vi "Get Display Data.vi"(7 "Filter Configuration Array":refnum<class "Base Filter.lvclass">[](array[class]), 8 "error in (no error)":errorcluster, 11 "Standard Display Configuration in":refnum<class "Standard Display Configuration.lvclass">) -> (0 "error out":errorcluster, 2 "Display Data":T1)   [LabVIEW 2018, in "Assert API Components.lvlib" / "Assert Display.lvlib" / "Main Display.lvlib" / "Standard Display Configuration.lvclass"]
uses:
  Standard Display Configuration.lvclass
  C:/Users/UKHornP/Documents/Work/Projects/Assert API/Core/Main Display/Display Configurations/Base Display Configuration.lvclass
  Components/Display Data.ctl
  Main Display/Display Colours.ctl
  Assert API Components/Filter Configurations/Base Filter.lvclass
  Base Display Configuration.lvclass/Base Display Configuration.ctl
  Base Display Configuration.lvclass
  Main Display.lvlib
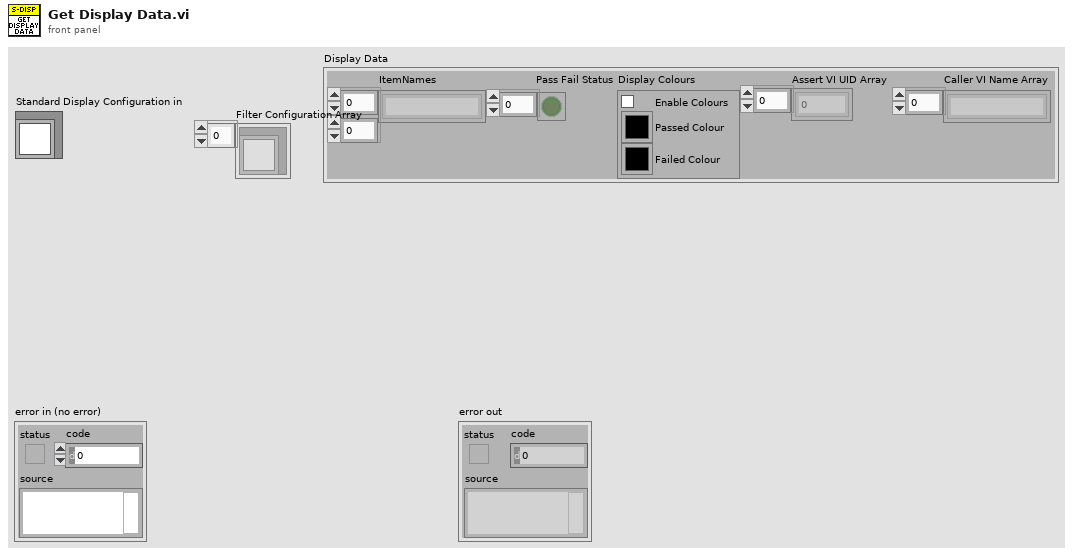
[diagram p1: front panel]
types:
  T1 = typedef "Assert API Components.lvlib/Assert Display.lvlib/Main Display.lvlib/Display Data.ctl" = cluster{"ItemNames":string[][], "Pass Fail Status":bool[], "Display Colours":T2, "Assert VI UID Array":i32[], "Caller VI Name Array":string[]}
  T2 = typedef "Assert API Components.lvlib/Assert Display.lvlib/Main Display.lvlib/Display Colours.ctl" = cluster{"Enable Colours":bool, "Passed Colour":u32, "Failed Colour":u32}
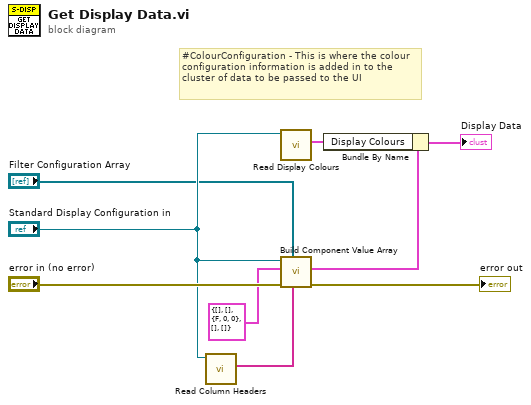
[diagram p0: block diagram]
diagram:
  # "#ColourConfiguration - This is where the colour configuration information is added in to the cluster of data to be passed to the UI"
  n1 = call "Read Column Headers.vi"("Base Display Configuration in"="Standard Display Configuration in") -> ("Column Headers"=w1:string[])  [unwired: 10 in]
  n2 = call "Read Display Colours.vi"("Base Display Configuration in"="Standard Display Configuration in") -> ("Display Colours"=w5:T2)  [unwired: 10 in]
  n3 = call "Build Component Value Array.vi"("Component Name Array"=w1, "Filter Configuration Array"="Filter Configuration Array", "error in (no error)"="error in (no error)", "Display Data in"=T1 {"ItemNames"=[], "Pass Fail Status"=[], "Display Colours"={"Enable Colours"=FALSE, "Passed Colour"=0, "Failed Colour"=0}, "Assert VI UID Array"=[], "Caller VI Name Array"=[]} ("Display Data"), "Standard Display Configuration in"="Standard Display Configuration in") -> ("error out"=→"error out":errorcluster, "Display Data out"=w3:T1)  [unwired: 5 in]
  n4 = Bundle By Name(cluster=w3, "Display Colours"=w5) -> (→"Display Data":T1)
